vi "Initialize.vi"(8 "error in (no error)":errorcluster, 9 "Reset (True)":bool=TRUE, 10 "ID Query (True)":bool=TRUE, 11 "VISA resource name":refnum<visa-resource-name>) -> (0 "error out":errorcluster, 3 "VISA resource name out":refnum<visa-resource-name>)   [LabVIEW 2017, in "Agilent E4980.lvlib"]
doc: "Establishes communication with the instrument and optionally performs an instrument identification query and/or an instrument reset. It also places the instrument in a default state needed for other instrument driver operations. Therefore, call this VI before calling other instrument driver VIs for this instrument. Generally, you need to call the Initialize VI only once at the beginning of an application."
uses:
  Agilent E4980.lvlib
  <vilib>/regexp/Match Regular Expression.xnode
panel:
  # "(c) 2007-2015 National Instruments.  ALL RIGHTS RESERVED."
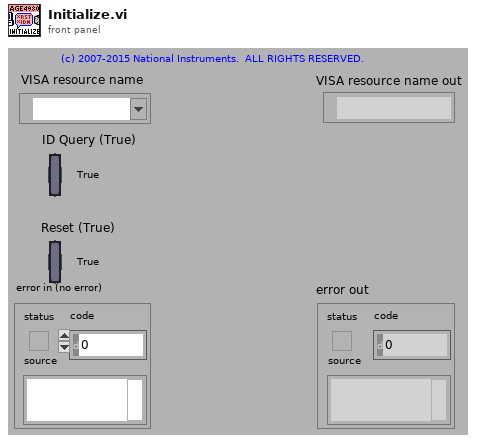
[diagram p1: front panel]
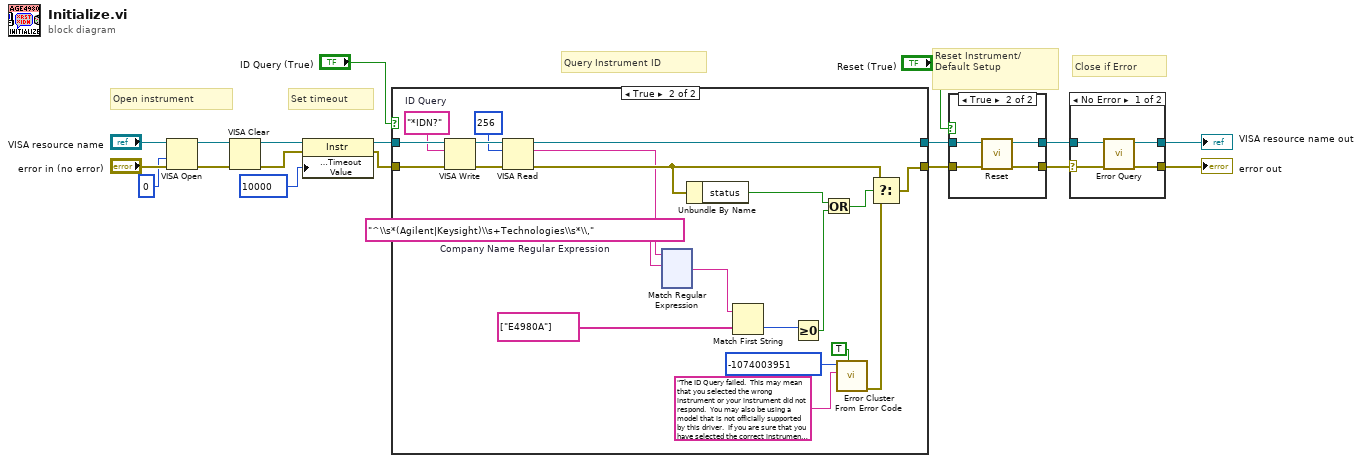
[diagram p0: block diagram]
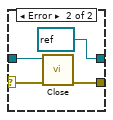
[diagram p2: hidden frame]
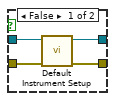
[diagram p3: hidden frame]
diagram:
  # "Set timeout"
  # "Close if Error"
  # "Query Instrument ID"
  # "Reset Instrument/\nDefault Setup"
  # "Open instrument"
  n1 = VISA Open(access mode=u32 0, error in (no error)="error in (no error)", VISA resource name="VISA resource name") -> (VISA resource name=w10:refnum<visa-resource-name>, error out=w9:errorcluster)  [unwired: 2 in]
  n2 = VISA Clear(VISA resource name=w10, error in (no error)=w9) -> (VISA resource name out=w8:refnum<visa-resource-name>, error out=w7:errorcluster)
  n3 = property class="Instr"(reference=w8, error in=w7, "General Settings:Timeout Value"=u32 10000) -> (reference out=w2:refnum<visa-resource-name>, error out=w1:errorcluster)
  n4 = case shown="True" "ID Query (True)" {
    tunnel: [w19 w41] -> w17
    tunnel: [w20 w38] -> w18
    tunnel: w2 -> [w20 w39]
    tunnel: w1 -> [w19 w40]
    frame False {
    }
    frame True {
      w22 = "^\\s*(Agilent|Keysight)\\s+Technologies\\s*\\,"  # Company Name Regular Expression
      w34 = "*IDN?"  # ID Query
      n5 = VISA Write(VISA resource name=w39, write buffer=w34, error in (no error)=w40) -> (VISA resource name out=w37:refnum<visa-resource-name>, error out=w36:errorcluster)  [unwired: 1 out]
      n6 = VISA Read(VISA resource name=w37, byte count=u32 256, error in (no error)=w36) -> (VISA resource name out=w38:refnum<visa-resource-name>, read buffer=w23:string, error out=w28:errorcluster)  [unwired: 1 out]
      n7 = xnode "Match Regular Expression"("input string"=w23, "regular expression"=w22) -> ("after match"=w21:string)  [unwired: 4 in, 4 out]
      n8 = Unbundle By Name(w28) -> ("status"=w27:bool)
      n9 = Match First String(2:string[] ["E4980A"] ("string array"), 3:w21) -> (0:w29:i32)  [unwired: 1 out]
      n10 = Greater Or Equal To 0?(x=w29) -> (x >= 0?=w26:bool)
      n11 = Or(x=w27, y=w26) -> (x .or. y?=w25:bool)
      n12 = call <vilib>:"Error Cluster From Error Code.vi"("show call chain? (False)"=TRUE, "error message (\"\")"="The ID Query failed.  This may mean that you selected the wrong instrument or your instrument did not respond.  You may also be using a model that is not officially supported by this driver.  If you are sure that you have selected the correct instrument and it is responding, try disabling the ID Query." ("Source (VI Name)"), "error code (0)"=-1074003951 ("Code")) -> ("error out"=w33:errorcluster)  [unwired: 6 in]
      n13 = Select(t=w28, s=w25, f=w33) -> (s? t:f=w41:errorcluster)
    }
  }
  n14 = case shown="True" "Reset (True)" {
    tunnel: w17 -> [w158 w160]
    tunnel: [w157 w163] -> w3
    tunnel: w18 -> [w159 w161]
    tunnel: [w156 w162] -> w4
    frame False {
      n15 = call "Default Instrument Setup.vi"("error in (no error)"=w158, "VISA resource name"=w159) -> ("error out"=w157:errorcluster, "VISA resource name out"=w156:refnum<visa-resource-name>)  [unwired: 8 in]
    }
    frame True {
      n16 = call "Reset.vi"("error in (no error)"=w160, "VISA resource name"=w161) -> ("error out"=w163:errorcluster, "VISA resource name out"=w162:refnum<visa-resource-name>)  [unwired: 8 in]
    }
  }
  n17 = case shown="No Error" w3 {
    selector: w3 -> [w165 w169]
    tunnel: w4 -> [w164 w170]
    tunnel: [w167 refnum<visa-resource-name> refnum ("VISA resource name out")] -> w6
    tunnel: [w166 w171] -> w5
    frame No Error {
      n18 = call "Error Query.vi"("error in (no error)"=w165, "VISA resource name"=w164) -> ("error out"=w166:errorcluster, "VISA resource name out"=w167:refnum<visa-resource-name>)  [unwired: 6 in, 2 out]
    }
    frame Error {
      n19 = call "Close.vi"("error in (no error)"=w169, "VISA resource name"=w170) -> ("error out"=w171:errorcluster)  [unwired: 9 in]
    }
  }
  "VISA resource name out" <- w6
  "error out" <- w5
